vi "exec.vi"(8 "error in (no error)":errorcluster, 10 "context":refnum<class "Context.lvclass">, 11 "StopMotion in":refnum<class "StopMotion.lvclass">) -> (0 "error out":errorcluster, 2 "context 2":refnum<class "Context.lvclass">, 3 "StopMotion out":refnum<class "StopMotion.lvclass">)   [LabVIEW 2015, in "StopMotion.lvclass"]
uses:
  StopMotion.lvclass
  Context/Context.lvclass
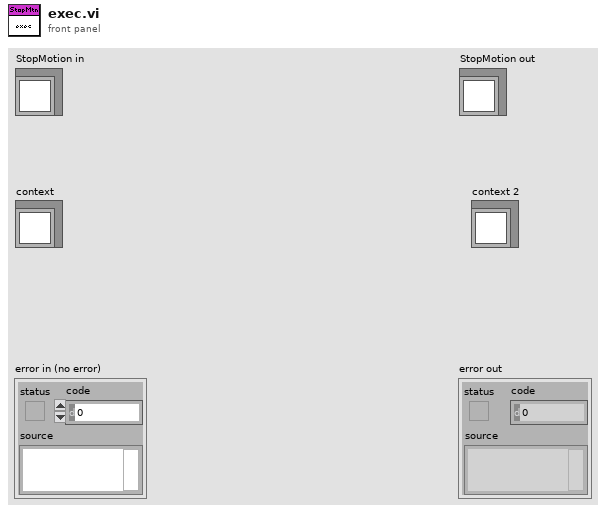
[diagram p1: front panel]
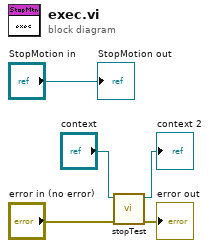
[diagram p0: block diagram]
diagram:
  n1 = call "stopTest.vi"("error in (no error)"="error in (no error)", "Context in"="context") -> ("error out"=→"error out":errorcluster, "Context out"=→"context 2":refnum<class "Context.lvclass">)  [unwired: 8 in]
  "StopMotion out" <- "StopMotion in"
